vi "Write Enabled.vi"(8 "error in (no error)":errorcluster, 10 "Enabled":bool=TRUE, 11 "MenuItem in":refnum<class "MGI_MenuItem.lvclass">) -> (0 "error out":errorcluster, 3 "MenuItem out":refnum<class "MGI_MenuItem.lvclass">)   [LabVIEW 2016, in "MGI_MenuItem.lvclass"]
doc: "Authored by Derek E. Trepanier\nsupport@mooregoodideas.com\nwww.mooregoodideas.com\n\nCopyright (c) 2012, Moore Good Ideas, Inc.\n\nAll rights reserved.\n\nRedistribution and use in source and binary forms, with or without modification, are permitted provided that the following conditions are met:\n\n * Redistributions of source code must retain the above copyright notice, this list of conditions and the following disclaimer.\n * Redistributions in binary form must reproduce the above copyright notice, this list of conditions and the following disclaimer in the documentation and/or other materials provided with the distribution.\n * Neither the name of Moore Good Ideas, Inc. nor the names of its contributors may be used to endorse or promote products derived from this software without specific prior written permission.\n\nTHIS SOFTWARE IS PROVIDED BY THE COPYRIGHT HOLDERS AND CONTRIBUTORS \"AS IS\" AND ANY EXPRESS OR IMPLIED WARRANTIES, INCLUDING, BUT NOT LIMITED TO, THE IMPLIED WARRANTIES OF MERCHANTABILITY AND FITNESS FOR A PARTICULAR PURPOSE ARE DISCLAIMED. IN NO EVENT SHALL THE COPYRIGHT OWNER OR CONTRIBUTORS BE LIABLE FOR ANY DIRECT, INDIRECT, INCIDENTAL, SPECIAL, EXEMPLARY, OR CONSEQUENTIAL DAMAGES (INCLUDING, BUT NOT LIMITED TO, PROCUREMENT OF SUBSTITUTE GOODS OR SERVICES; LOSS OF USE, DATA, OR PROFITS; OR BUSINESS INTERRUPTION) HOWEVER CAUSED AND ON ANY THEORY OF LIABILITY, WHETHER IN CONTRACT, STRICT LIABILITY, OR TORT (INCLUDING NEGLIGENCE OR OTHERWISE) ARISING IN ANY WAY OUT OF THE USE OF THIS SOFTWARE, EVEN IF ADVISED OF THE POSSIBILITY OF SUCH DAMAGE."
uses:
  <userlib>/_MGI/Menu Building/MenuItem/MGI_MenuItem.lvclass
  <userlib>/_MGI/Menu Building/MenuItem/MGI_MenuItem.lvclass/MGI_MenuItem.ctl
  <userlib>/_MGI/Menu Building/MenuTypes/MGI_Menu.lvclass
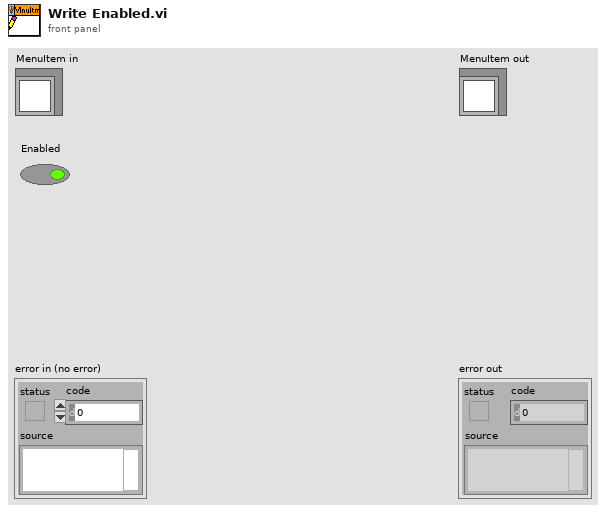
[diagram p1: front panel]
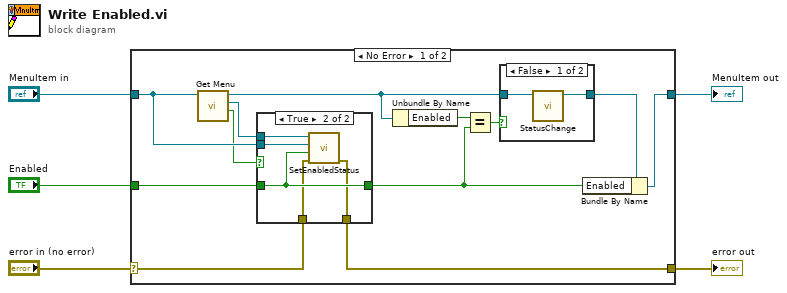
[diagram p0: block diagram]
diagram:
  n1 = case shown="No Error" "error in (no error)" {
    selector: "error in (no error)" -> [w12 w28]
    tunnel: [w11 w28] -> w4
    tunnel: [w17 w29] -> w2
    tunnel: "MenuItem in" -> [w15 w29]
    tunnel: "Enabled" -> [w14 _]
    frame No Error {
      n2 = call <userlib>:"Get Menu.vi"("MenuItem in"=w15) -> ("Menu Valid"=w13:bool, "Menu"=w16:refnum<class "MGI_Menu.lvclass">, "MenuItem out"=w8:refnum<class "MGI_MenuItem.lvclass">)  [unwired: 7 in, 1 out]
      n3 = case shown="True" w13 {
        tunnel: w16 -> [_ w27]
        tunnel: w15 -> [_ w26]
        tunnel: w14 -> [w22 w25]
        tunnel: [w22 w25] -> w6
        tunnel: w12 -> [w21 w24]
        tunnel: [w21 w23] -> w11
        frame False {
        }
        frame True {
          n4 = call-dynamic "SetEnabledStatus.vi"("error in (no error)"=w24, "Enabled"=w25, "MenuItem"=w26, "Menu in"=w27) -> ("error out"=w23:errorcluster)  [unwired: 6 in, 1 out]
        }
      }
      n5 = Unbundle By Name(w8) -> ("Enabled"=w7:bool)
      n6 = Equal?(x=w7, y=w6) -> (x = y?=w9:bool)
      n7 = case shown="False" w9 {
        tunnel: w8 -> [w19 w20]
        tunnel: [w18 w20] -> w10
        frame False {
          n8 = call-dynamic "StatusChange.vi"("MGI_MenuItem in"=w19) -> ("MGI_MenuItem out"=w18:refnum<class "MGI_MenuItem.lvclass">)  [unwired: 9 in, 1 out]
        }
        frame True {
        }
      }
      n9 = Bundle By Name(cluster=w10, "Enabled"=w6) -> (w17:refnum<class "MGI_MenuItem.lvclass">)
    }
    frame Error {
    }
  }
  "error out" <- w4
  "MenuItem out" <- w2
